vi "Configure Time Domain Display Range.vi"(0 "VISA resource name":refnum<visa-resource-name>, 1 "Channel (1)":i32=1, 2 "Setting Type  (1: Start / Stop)":u16(ring)=1 items=["Center/Span", "Start / Stop"], 5 "Start / Center (0.0)":dbl format="%^.2e", 7 "Stop / Span (10.0E-9)":dbl=1e-08 format="%^.2e", 11 "error in (no error)":errorcluster) -> (4 "VISA resource name out":refnum<visa-resource-name>, 15 "error out":errorcluster)   [LabVIEW 2018, in "Agilent ENA Series.lvlib"]
doc: "Configures time domain display range."
uses:
  Agilent ENA Series.lvlib
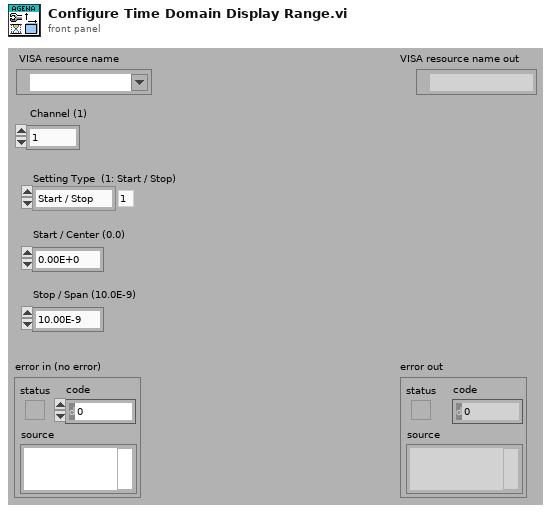
[diagram p1: front panel]
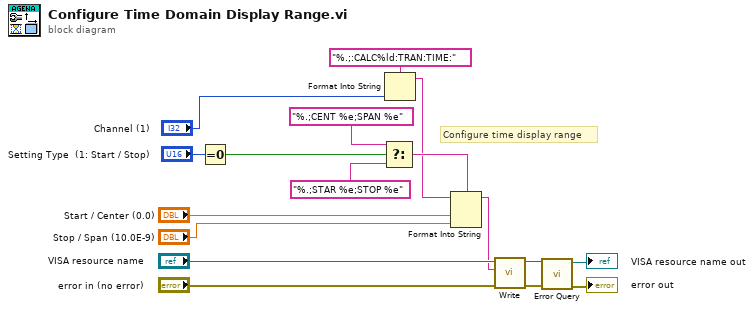
[diagram p0: block diagram]
diagram:
  # "Configure time display range"
  n1 = Equal To 0?(x="Setting Type  (1: Start / Stop)") -> (x = 0?=w12:bool)
  n2 = Select(t="%.;CENT %e;SPAN %e", s=w12, f="%.;STAR %e;STOP %e") -> (s? t:f=w9:string)
  n3 = Format Into String(format string="%.;:CALC%ld:TRAN:TIME:", "Channel (1)") -> (resulting string=w6:string)  [unwired: 2 in, 1 out]
  n4 = Format Into String(format string=w9, initial string=w6, "Start / Center (0.0)", "Stop / Span (10.0E-9)") -> (resulting string=w5:string)  [unwired: 1 in, 1 out]
  n5 = call "Write.vi"("error in (no error)"="error in (no error)", "String ()"=w5, "VISA resource name"="VISA resource name") -> ("error out"=w3:errorcluster, "VISA resource name out"=w4:refnum<visa-resource-name>)  [unwired: 6 in, 1 out]
  n6 = call "Error Query.vi"("error in (no error)"=w3, "VISA resource name"=w4) -> ("error out"=→"error out":errorcluster, "VISA resource name out"=→"VISA resource name out":refnum<visa-resource-name>)  [unwired: 6 in, 2 out]
